vi "Acquire_nodt.vi"(0 "Ch Armed Reg":refnum<k21>="Register 1", 1 "Command FIFO":refnum<k21>, 3 "Circular Buffer Mem":refnum<k21>, 4 "circular buffer length":u32=300, 5 "FPGA I/O In":refnum<k21>="IO Module\\AI A0", 7 "channel on/off":bool, 9 "Trigger":i16=1500, 10 "Timing FIFO":refnum<k21>, 11 "Samples to Acquire":u32=100, 14 "# of pretrigger":u32=15, 15 "timing":u64) -> ()   [LabVIEW 2012]
uses:
  <vilib>/rvi/DataTransferAndStorage/Container/XNode/niFpgaContainer.xnode
  <vilib>/eio/EIONode/EIONode.xnode
  <vilib>/rvi/DataTransferAndStorage/Register/Emulation/niFpgaRegisterEmulationRefIn.vi
  <vilib>/rvi/FIFO/Fifo_Resource/niFpgaFifoEmulationRefIn.vi
  <vilib>/rvi/eio/common/nirviEmuTemplateMethod_errors.vi
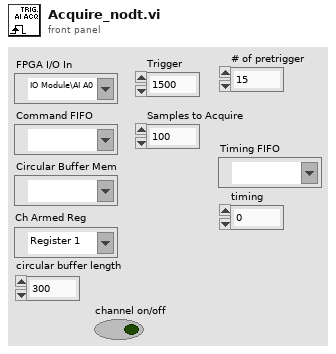
[diagram p1: front panel]
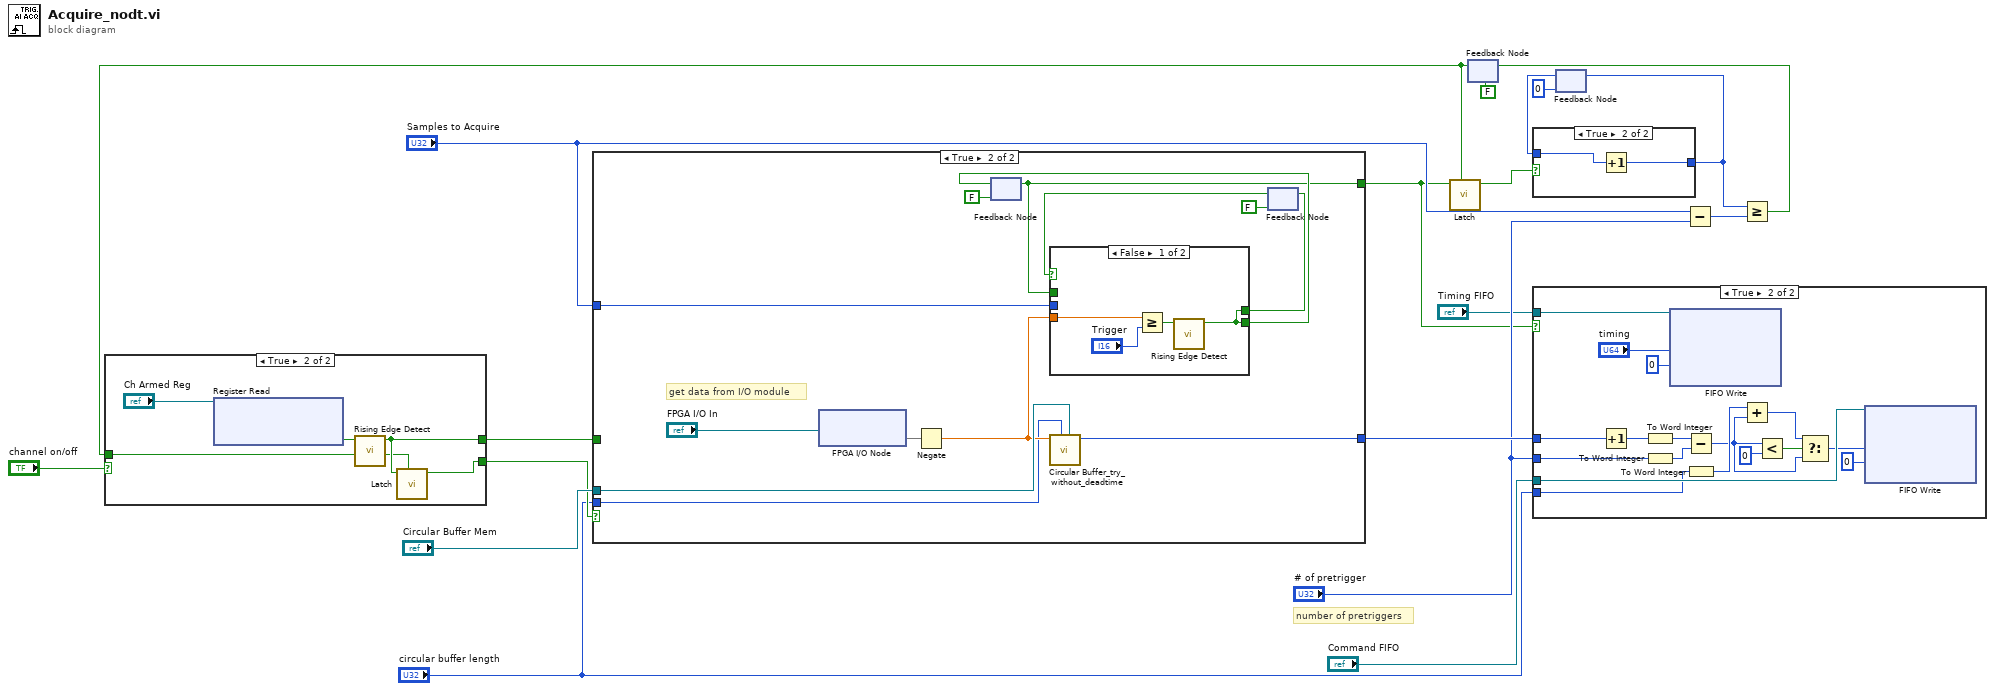
[diagram p0: block diagram]
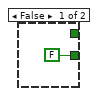
[diagram p2: hidden frame]
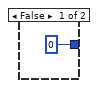
[diagram p3: hidden frame]
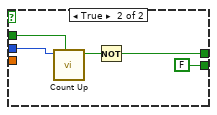
[diagram p5: hidden frame]
diagram:
  # "number of pretriggers"
  n1 = feedback #1(FALSE) -> (w1:bool)
  n2 = case shown="True" "channel on/off" {
    tunnel: [FALSE ("Output") w23] -> w16
    tunnel: [_ w22] -> w15
    tunnel: w1 -> [_ w21]
    frame False {
    }
    frame True {
      n3 = xnode ("Register Read")("Register In"="Ch Armed Reg") -> ("Data"=w24:bool)  [unwired: 1 out]
      n4 = call "Rising Edge Detect.vi"("Input"=w24) -> ("Rising Edge"=w22:bool)  [unwired: 10 in]
      n5 = call "Latch.vi"("Reset"=w21, "Input"=w22) -> ("Output"=w23:bool)  [unwired: 9 in]
    }
  }
  n6 = case shown="True" w16 {
    tunnel: "Circular Buffer Mem" -> [_ w38]
    tunnel: "circular buffer length" -> [_ w36]
    tunnel: [_ w35] -> w17
    tunnel: w15 -> [_ _]
    tunnel: "Samples to Acquire" -> [_ w31]
    tunnel: [_ w29] -> w2
    frame False {
    }
    frame True {
      # "get data from I/O module"
      n7 = xnode "FPGA I/O Node"("FPGA I/O In"="FPGA I/O In") -> ("I/O Item"=w27)  [unwired: 1 out]
      n8 = Negate(x=w27) -> (-x=w37:dbl)
      n9 = feedback #2(FALSE ("Rising Edge")) -> (w29:bool)
      n10 = call "Circular Buffer_try_without_deadtime.vi"("Refnum in"=w38, "circular buffer length"=w36, "Data"=w37) -> ("Address"=w35:u16)  [unwired: 8 in]
      n11 = feedback #3(FALSE ("Rising Edge")) -> (w34:bool)
      n12 = case shown="False" w34 {
        tunnel: w37 -> [w42 _]
        tunnel: [w39 w45] -> w32
        tunnel: w31 -> [_ w47]
        tunnel: [w39 FALSE ("Rising Edge")] -> w30
        tunnel: w29 -> [_ w44]
        frame False {
          n13 = Greater Or Equal?(x=w42, y="Trigger") -> (x >= y?=w40:bool)
          n14 = call "Rising Edge Detect.vi"("Input"=w40) -> ("Rising Edge"=w39:bool)  [unwired: 10 in]
        }
        frame True {
          n15 = call "Count Up.vi"("Reset?"=w44, "goal"=w47) -> ("Count Met"=w46:bool)  [unwired: 8 in, 1 out]
          n16 = Not(x=w46) -> (.not. x?=w45:bool)
        }
      }
      n17 = feedback-in #2(w30) -> ()
      n18 = feedback-in #3(w32) -> ()
    }
  }
  n19 = call "Latch.vi"("Reset"=w1, "Input"=w2) -> ("Output"=w12:bool)  [unwired: 9 in]
  n20 = case shown="True" w2 {
    tunnel: "Command FIFO" -> [_ w64]
    tunnel: w17 -> [_ w49]
    tunnel: "# of pretrigger" -> [_ w50]
    tunnel: "circular buffer length" -> [_ w48]
    tunnel: "Timing FIFO" -> [_ w62]
    frame False {
    }
    frame True {
      n21 = Increment(x=w49) -> (x+1=w57:u16)
      n22 = To Word Integer(number=w57) -> (16bit integer=w58:i16)
      n23 = To Word Integer(number=w50) -> (16bit integer=w59:i16)
      n24 = xnode ("FIFO Write")("Element"="timing", "Timeout"=0, "FIFO In"=w62) -> ()  [unwired: 2 out]
      n25 = Subtract(x=w58, y=w59) -> (x-y=w55:i16)
      n26 = To Word Integer(number=w48) -> (16bit integer=w56:i16)
      n27 = Add(x=w56, y=w55) -> (x+y=w54:i16)
      n28 = Less?(x=w55, y=i16 0) -> (x < y?=w52:bool)
      n29 = Select(t=w54, s=w52, f=w55) -> (s? t:f=w51:i16)
      n30 = xnode ("FIFO Write")("Element"=w51, "Timeout"=0, "FIFO In"=w64) -> ()  [unwired: 2 out]
    }
  }
  n31 = feedback #4(u32 0) -> (w8:u32)
  n32 = case shown="True" w12 {
    tunnel: [u32 0 w67] -> w6
    tunnel: w8 -> [_ w66]
    frame False {
    }
    frame True {
      n33 = Increment(x=w66) -> (x+1=w67:u32)
    }
  }
  n34 = feedback-in #4(w6) -> ()
  n35 = Subtract(x="Samples to Acquire", y="# of pretrigger") -> (x-y=w11:u32)
  n36 = Greater Or Equal?(x=w6, y=w11) -> (x >= y?=w10:bool)
  n37 = feedback-in #1(w10) -> ()
